vi "2013-05-07_circle.vi"() -> ()   [LabVIEW 2020]
panel:
  out "1-bit pixmap":bool[][](array[boolean]) caption="1-Bit-Pixmap"
  in  "radius":i16 caption="Radius"
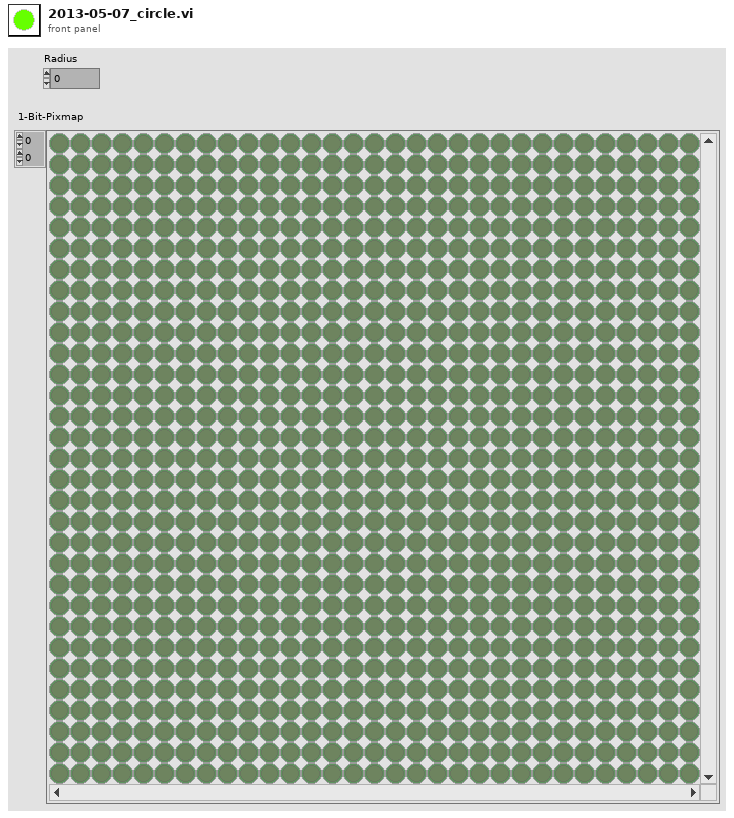
[diagram p1: front panel]
types:
  T1 = typedef "imagedata.ctl" = cluster{"image type":i32, "image depth":i32, "image":u8[], "mask":u8[], "colors":u32[], "Rectangle":cluster{"left":i16, "top":i16, "right":i16, "bottom":i16}}
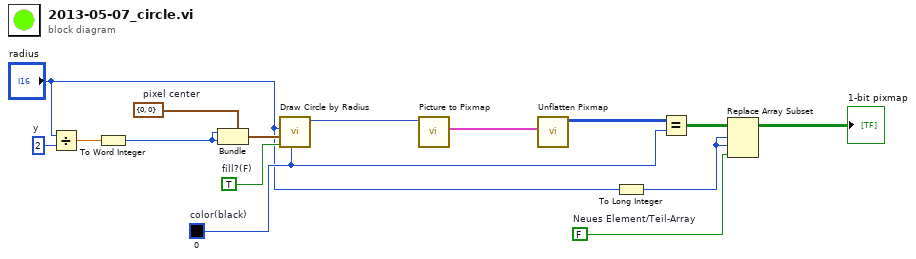
[diagram p0: block diagram]
diagram:
  w4 = FALSE  # Neues Element/Teil-Array
  w7 = u32 0  # color(black)
  w11 = TRUE  # fill?(F)
  w13 = cluster{"horizontal":i16, "vertical":i16} {"horizontal"=0, "vertical"=0}  # pixel center
  w15 = i16 2  # y
  n1 = Divide(x="radius", y=w15) -> (x/y=w14:dbl)
  n2 = To Word Integer(number=w14) -> (16bit integer=w5:i16)
  n3 = Bundle "Bundle"(cluster=w13, "horizontal"=w5, "vertical"=w5) -> (w12:cluster{"horizontal":i16, "vertical":i16})
  n4 = call <vilib>:"Draw Circle by Radius.vi"("color(black)"=w7, "fill?(F)"=w11, "pixel center"=w12, "radius"="radius") -> ("new picture"=w10:picture)  [unwired: 7 in]
  n5 = call <vilib>:"Picture to Pixmap.vi"("picture"=w10) -> ("image data"=w9:T1)  [unwired: 9 in, 1 out]
  n6 = call <vilib>:"Unflatten Pixmap.vi"("image data"=w9) -> ("24-bit pixmap"=w8:u32[][])  [unwired: 4 in, 6 out]
  n7 = To Long Integer(number="radius") -> (32bit integer=w1:i32)
  n8 = Equal?(x=w8, y=w7) -> (x = y?=w6:bool[][])
  n9 = Replace Array Subset "Replace Array Subset"(array=w6, new element=w4, index (row)=w1, index (col)=w1) -> (→"1-bit pixmap":bool[][])
